vi "trash_Refresh Stats Command.vi"(8 "error in":errorcluster, 11 "CoreOOB_Rx in":refnum<class "ChanMngOOB_Rx.lvclass">) -> (0 "error out":errorcluster, 3 "CoreOOB_Rx out":refnum<class "ChanMngOOB_Rx.lvclass">)   [LabVIEW 2021]
uses:
  ChanMngOOB_Rx.lvclass/ChanMngOOB_Rx.ctl
  Typedef/OOB ChnMng Commands.ctl
  ChanMngOOB_Rx.lvclass
  <vilib>/CIF Foundation/CIF Out of Band Commands/Typedef/OOB Container.ctl
  <vilib>/CIF Foundation/CIF Out of Band Commands/CIFOutOfBand.lvclass
  C:/Program Files/National Instruments/LabVIEW 2021/vi.lib/CIF Foundation/CIF Out of Band Commands/CIFOutOfBand.lvclass
  D:/dev/CIF-LVCore/src/Channels/CIFChannelMng/OOB/OOB_Rx/ChanMngOOB_Rx.lvclass
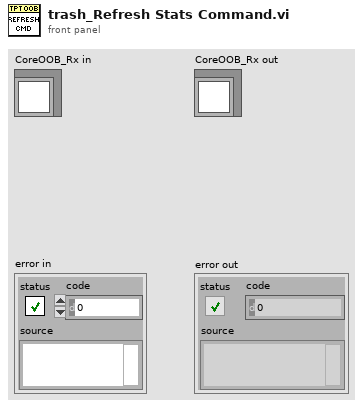
[diagram p1: front panel]
types:
  T1 = typedef "CIFOutOfBand.lvclass/OOB Container.ctl" = cluster{"Commands (bitwise)":u64, "Payload":variant}
  T2 = typedef "ChanMngOOB_Rx.lvclass/OOB ChnMng Commands.ctl" = enum8{"Start", "Pause", "Stop", "RefreshStats", "UpdateConfig", "Connect Channel", "Force Channel", "Update Clock Map"}
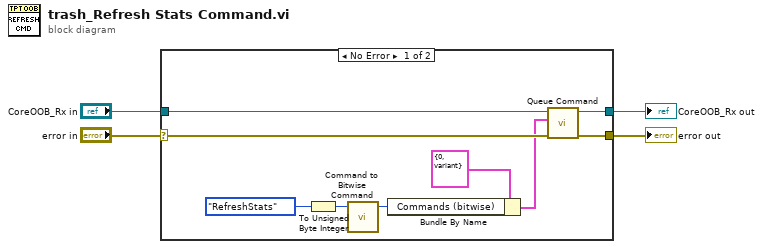
[diagram p0: block diagram]
diagram:
  n1 = case shown="No Error" "error in" {
    selector: "error in" -> [w11 w15]
    tunnel: [w12 w15] -> w1
    tunnel: "CoreOOB_Rx in" -> [w10 w14]
    tunnel: [w13 w14] -> w2
    frame No Error {
      n2 = To Unsigned Byte Integer(number=OOB_ChnMng_Commands."RefreshStats" ("OOB Main Commands")) -> (unsigned 8bit integer=w9:u8)
      n3 = call <vilib>:"Command to Bitwise Command.vi"("Command"=w9) -> ("bit command"=w6:u64)  [unwired: 3 in]
      n4 = Bundle By Name(cluster=T1 {"Commands (bitwise)"=0, "Payload"=variant} ("OOB Data"), "Commands (bitwise)"=w6) -> (w5:T1)
      n5 = call <vilib>:"Queue Command.vi"("error in"=w11, "OOB Data"=w5, "OOB in"=w10) -> ("error out"=w12:errorcluster, "OOB out"=w13:refnum<class "ChanMngOOB_Rx.lvclass">)  [unwired: 7 in]
    }
    frame Error {
    }
  }
  "error out" <- w1
  "CoreOOB_Rx out" <- w2
